vi "U6 Quadrature Read.vi"(8 "error in":errorcluster, 9 "Reset Count":bool, 10 "Timer #":u8, 11 "Handle In":i32) -> (0 "error out":errorcluster, 1 "Quadrature Count":i32, 3 "Handle Out":i32)   [LabVIEW 2021]
panel:
  out "Error Message":string
  # "Reads from an already configured quadrature input."
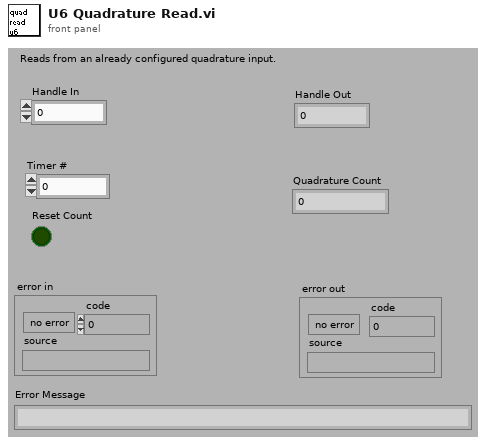
[diagram p1: front panel]
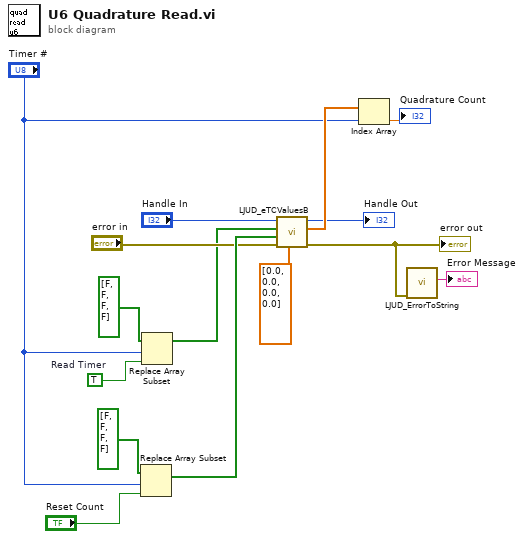
[diagram p0: block diagram]
diagram:
  w3 = TRUE  # Read Timer
  n1 = Replace Array Subset(array=bool[] [FALSE, FALSE, FALSE, FALSE] ("aUpdateResetTimers"), new element="Reset Count", index="Timer #") -> (w9:bool[])
  n2 = Replace Array Subset(array=bool[] [FALSE, FALSE, FALSE, FALSE] ("aUpdateResetTimers"), new element=w3, index="Timer #") -> (w2:bool[])
  n3 = call "LJUD_eTCValuesB.vi"("aTimerValues Write"=dbl[] [0.0, 0.0, 0.0, 0.0], "error in"="error in", "aUpdateResetTimers"=w9, "aReadTimers"=w2, "Handle In"="Handle In") -> ("error out"=w8:errorcluster, "aTimerValues Read"=w13:dbl[], "Handle Out"=→"Handle Out":i32)  [unwired: 3 in, 1 out]
  "error out" <- w8
  n4 = Index Array(array=w13, index="Timer #") -> (element=→"Quadrature Count":dbl)
  n5 = call "LJUD_ErrorToString.vi"("error in"=w8) -> ("String"=→"Error Message":string)  [unwired: 10 in]
